vi "Read Force Measured.vi"(11 "ForceSensor in":refnum<class "ForceSensorCalculator.lvclass">) -> (2 "Force Demand":dbl[unit] min=-888.0 max=888.0 format="%.2f", 3 "ForceSensor out":refnum<class "ForceSensorCalculator.lvclass">)   [LabVIEW 2013, in "ForceSensorCalculator.lvlib" / "ForceSensorCalculator.lvclass"]
uses:
  <userlib>/Common/Devices/ForceSensorCalculator/ForceSensorCalculator/ForceSensorCalculator.lvclass
  <userlib>/Common/Devices/ForceSensorCalculator/ForceSensorCalculator/ForceSensorCalculator.lvclass/ForceSensorCalculator.ctl
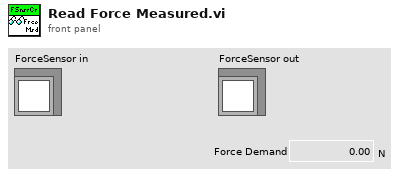
[diagram p1: front panel]
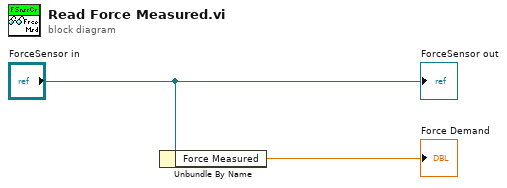
[diagram p0: block diagram]
diagram:
  n1 = Unbundle By Name("ForceSensor in") -> ("Force Measured"=→"Force Demand":dbl[unit])
  "ForceSensor out" <- "ForceSensor in"
